vi "Init.vi"(8 "error in":errorcluster, 10 "Sourcegrid Container":refnum<k24>(container), 11 "PDO Grid in":refnum<class "PDO Grid.lvclass">) -> (0 "error out":errorcluster, 3 "PDO Grid out":refnum<class "PDO Grid.lvclass">)   [LabVIEW 2024, in "PDO Grid.lvlib" / "PDO Grid.lvclass"]
uses:
  PDO Grid/PDO Grid.lvclass
  D:/git/Sourcegrid-LabVIEW/source/Grid/SourceGrid.lvclass
  PDO Mapping ColumnHeader/PDO Mapping ColumnHeader.lvclass
  D:/git/Sourcegrid-LabVIEW/source/Cells/Cell/Cell.lvclass
  Sourcegrid-LabVIEW/source/System.Drawing.Color.ctl
  Sourcegrid-LabVIEW/source/Grid/Set FixedRows.vi
  Sourcegrid-LabVIEW/source/Grid/Set SelectionMode.vi
  Sourcegrid-LabVIEW/source/Grid/SourceGrid.lvclass
  PDO Grid/PDO Grid.lvclass/PDO Grid.ctl
  D:/git/Sourcegrid-LabVIEW/dll/SourceGrid.dll
  Sourcegrid-LabVIEW/dll/SourceGrid.dll
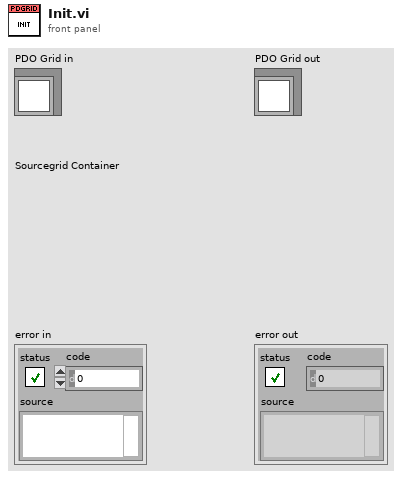
[diagram p1: front panel]
types:
  T1 = typedef "System.Drawing.Color.ctl" = enum16{"AliceBlue", "AntiqueWhite", "Aqua", "Aquamarine", "Azure", "Beige", "Bisque", "Black", "BlanchedAlmond", "Blue", "BlueViolet", "Brown", "BurlyWood", "CadetBlue", "Chartreuse", "Chocolate", "Coral", "CornflowerBlue", "Cornsilk", "Crimson", "Cyan", "DarkBlue", "DarkCyan", "DarkGoldenrod", "DarkGray", "DarkGreen", "DarkKhaki", "DarkMagenta", "DarkOliveGreen", "DarkOrange", "DarkOrchid", "DarkRed", "DarkSalmon", "DarkSeaGreen", "DarkSlateBlue", "DarkSlateGray", "DarkTurquoise", "DarkViolet", "DeepPink", "DeepSkyBlue", "DimGray", "DodgerBlue", "Firebrick", "FloralWhite", "ForestGreen", "Fuchsia", "Gainsboro", "GhostWhite", "Gold", "Goldenrod", "Gray", "Green", "GreenYellow", "Honeydew", "HotPink", "IndianRed", "Indigo", "Ivory", "Khaki", "Lavender", "LavenderBlush", "LawnGreen", "LemonChiffon", "LightBlue", "LightCoral", "LightCyan", "LightGoldenrodYellow", "LightGray", "LightGreen", "LightPink", "LightSalmon", "LightSeaGreen", "LightSkyBlue", "LightSlateGray", "LightSteelBlue", "LightYellow", "Lime", "LimeGreen", "Linen", "Magenta", "Maroon", "MediumAquamarine", "MediumBlue", "MediumOrchid", "MediumPurple", "MediumSeaGreen", "MediumSlateBlue", "MediumSpringGreen", "MediumTurquoise", "MediumVioletRed", "MidnightBlue", "MintCream", "MistyRose", "Moccasin", "NavajoWhite", "Navy", "OldLace", "Olive", "OliveDrab", "Orange", "OrangeRed", "Orchid", "PaleGoldenrod", "PaleGreen", "PaleTurquoise", "PaleVioletRed", "PapayaWhip", "PeachPuff", "Peru", "Pink", "Plum", "PowderBlue", "Purple", "Red", "RosyBrown", "RoyalBlue", "SaddleBrown", "Salmon", "SandyBrown", "SeaGreen", "SeaShell", "Sienna", "Silver", "SkyBlue", "SlateBlue", "SlateGray", "Snow", "SpringGreen", "SteelBlue", "Tan", "Teal", "Thistle", "Tomato", "Transparent", "Turquoise", "Violet", "Wheat", "White", "WhiteSmoke", "Yellow"}
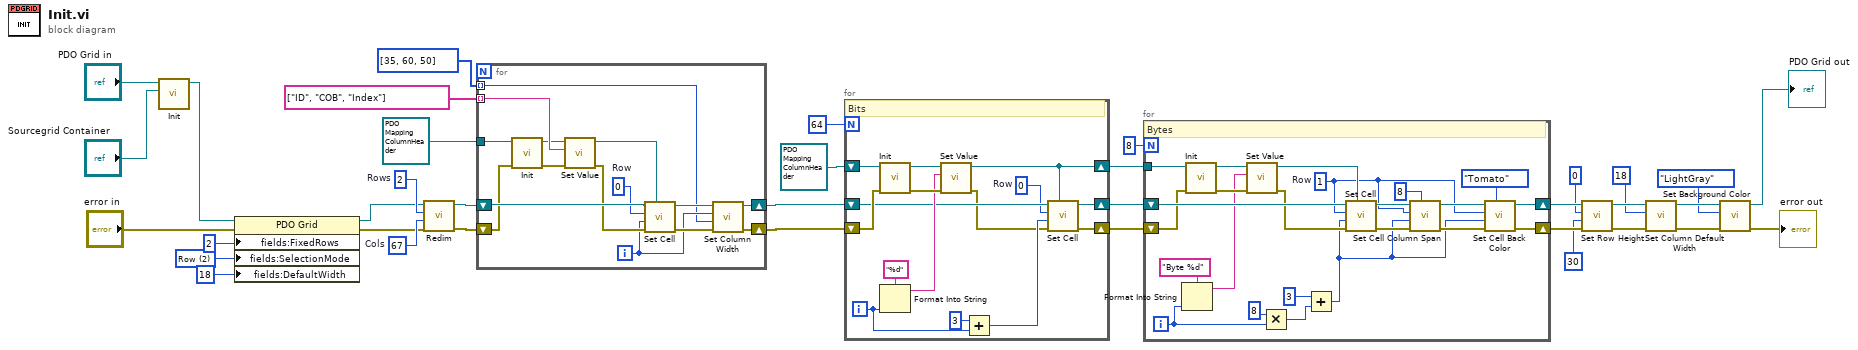
[diagram p0: block diagram]
diagram:
  w34 = 2 items=["Cell"=1, "Row"=2, "Column"=3] ("SelectionMode")
  w35 = 67  # Cols
  w36 = 2  # Rows
  n1 = call-parent "Init.vi"("Sourcegrid Container"="Sourcegrid Container", "Grid in"="PDO Grid in") -> ("Grid out"=w9:refnum<class "PDO Grid.lvclass">)  [unwired: 8 in, 1 out]
  n2 = property class="PDO Grid"(reference=w9, error in="error in", "fields:FixedRows"=2 ("FixedRows"), "fields:SelectionMode"=w34, "fields:DefaultWidth"=18 ("DefaultWidth")) -> (reference out=w28:refnum<class "PDO Grid.lvclass">, error out=w26:errorcluster)
  n3 = call "Redim.vi"("error in"=w26, "Columns"=w35, "Rows"=w36, "Sourcegrid in"=w28) -> ("error out"=w25:errorcluster, "Sourcegrid out"=w27:refnum<class "PDO Grid.lvclass">)  [unwired: 6 in]
  n4 = for {
    shift-right: [w45] -> w23
    shift-left: w25 -> [w48]
    shift-right: [w43] -> w22
    shift-left: w27 -> [w51]
    tunnel: string[] ["ID", "COB", "Index"] -> [w40] mode=indexing
    tunnel: refnum<class "PDO Mapping ColumnHeader.lvclass"> refnum ("UI Actor.lvlib:PDOMapping ColumnHeader.lvclass") -> [w38]
    tunnel: i32[] [35, 60, 50] -> [w41] mode=indexing
    i -> [w42]
    w49 = 0  # Row
    n5 = call-dynamic "Init.vi"("error in"=w48, "MyTestHeader in"=w38) -> ("error out"=w39:errorcluster, "MyTestHeader out"=w37:refnum<class "PDO Mapping ColumnHeader.lvclass">)  [unwired: 8 in]
    n6 = call-dynamic "Set Value.vi"("error in"=w39, "Value"=w40, "MyTestHeader in"=w37) -> ("error out"=w46:errorcluster, "MyTestHeader out"=w47:refnum<class "PDO Mapping ColumnHeader.lvclass">)  [unwired: 7 in]
    n7 = call "Set Cell.vi"("Cell"=w47, "error in"=w46, "Column"=w42, "Row"=w49, "Sourcegrid in"=w51) -> ("error out"=w50:errorcluster, "Sourcegrid out"=w44:refnum<class "PDO Grid.lvclass">)  [unwired: 5 in]
    n8 = call "Set Column Width.vi"("error in"=w50, "Width"=w41, "Column"=w42, "Sourcegrid in"=w44) -> ("error out"=w45:errorcluster, "Sourcegrid out"=w43:refnum<class "PDO Grid.lvclass">)  [unwired: 6 in]
  }
  n9 = for {
    N: 64 -> [_]
    shift-right: [w59] -> w13
    shift-left: w23 -> [w65]
    shift-right: [w58] -> w12
    shift-left: w22 -> [w57]
    shift-right: [w52] -> w2
    shift-left: refnum<class "PDO Mapping ColumnHeader.lvclass"> refnum ("UI Actor.lvlib:PDOMapping ColumnHeader.lvclass") -> [w53]
    i -> [w60]
    w56 = 0  # Row
    # "Bits"
    n10 = call-dynamic "Init.vi"("error in"=w65, "MyTestHeader in"=w53) -> ("error out"=w64:errorcluster, "MyTestHeader out"=w63:refnum<class "PDO Mapping ColumnHeader.lvclass">)  [unwired: 8 in]
    n11 = Format Into String(format string="%d", w60) -> (resulting string=w62:string)  [unwired: 2 in, 1 out]
    n12 = call-dynamic "Set Value.vi"("error in"=w64, "Value"=w62, "MyTestHeader in"=w63) -> ("error out"=w54:errorcluster, "MyTestHeader out"=w52:refnum<class "PDO Mapping ColumnHeader.lvclass">)  [unwired: 7 in]
    n13 = Add(x=3, y=w60) -> (x+y=w55:i32)
    n14 = call "Set Cell.vi"("Cell"=w52, "error in"=w54, "Column"=w55, "Row"=w56, "Sourcegrid in"=w57) -> ("error out"=w59:errorcluster, "Sourcegrid out"=w58:refnum<class "PDO Grid.lvclass">)  [unwired: 5 in]
  }
  n15 = for {
    N: 8 -> [_]
    shift-right: [w74] -> w21
    shift-left: w13 -> [w84]
    shift-right: [w72] -> w18
    shift-left: w12 -> [w88]
    tunnel: w2 -> [w67]
    i -> [w80]
    w69 = 1  # Row
    # "Bytes"
    n16 = Format Into String(format string="Byte %d", w80) -> (resulting string=w78:string)  [unwired: 2 in, 1 out]
    n17 = call-dynamic "Init.vi"("error in"=w84, "MyTestHeader in"=w67) -> ("error out"=w83:errorcluster, "MyTestHeader out"=w87:refnum<class "PDO Mapping ColumnHeader.lvclass">)  [unwired: 8 in]
    n18 = call-dynamic "Set Value.vi"("error in"=w83, "Value"=w78, "MyTestHeader in"=w87) -> ("error out"=w82:errorcluster, "MyTestHeader out"=w85:refnum<class "PDO Mapping ColumnHeader.lvclass">)  [unwired: 7 in]
    n19 = Multiply(x=8, y=w80) -> (x*y=w77:i32)
    n20 = Add(x=3, y=w77) -> (x+y=w68:i32)
    n21 = call "Set Cell.vi"("Cell"=w85, "error in"=w82, "Column"=w68, "Row"=w69, "Sourcegrid in"=w88) -> ("error out"=w89:errorcluster, "Sourcegrid out"=w76:refnum<class "PDO Grid.lvclass">)  [unwired: 5 in]
    n22 = call "Set Cell Column Span.vi"("Range"=8, "error in"=w89, "Column"=w68, "Row"=w69, "SourceGrid in"=w76) -> ("error out"=w71:errorcluster, "SourceGrid out"=w73:refnum<class "PDO Grid.lvclass">)  [unwired: 5 in]
    n23 = call "Set Cell Back Color.vi"("Color"=System.Drawing.Color."Tomato", "error in"=w71, "Column"=w68, "Row"=w69, "SourceGrid in"=w73) -> ("error out"=w74:errorcluster, "SourceGrid out"=w72:refnum<class "PDO Grid.lvclass">)  [unwired: 5 in]
  }
  n24 = call "Set Row Height.vi"("error in"=w21, "Height"=30, "Row"=0, "SourceGrid in"=w18) -> ("error out"=w19:errorcluster, "SourceGrid out"=w15:refnum<class "PDO Grid.lvclass">)  [unwired: 6 in]
  n25 = call "Set Column Default Width.vi"("error in"=w19, "Default Width"=18, "SourceGrid in"=w15) -> ("error out"=w11:errorcluster, "SourceGrid out"=w5:refnum<class "PDO Grid.lvclass">)  [unwired: 7 in]
  n26 = call "Set Background Color.vi"("error in"=w11, "Color"=System.Drawing.Color."LightGray", "SourceGrid in"=w5) -> ("error out"=→"error out":errorcluster, "SourceGrid out"=→"PDO Grid out":refnum<class "PDO Grid.lvclass">)  [unwired: 7 in]
